vi "Apply IMAQdx Attributes.vi"(8 "error in":errorcluster, 10 "<JSON>":string, 11 "IMAQdx Session in":T1) -> (0 "error out":errorcluster, 3 "Refnum out":T1)   [LabVIEW 2024, in "IMAQdx Base Configure Strategy.lvclass"]
uses:
  IMAQdx Base Configure Strategy.lvclass
  IMAQdx Base Configure Strategy.lvclass/IMAQdx Base Configure Strategy.ctl
  <resource>/objmgr/imaqdx.rc
  <vilib>/JDP Science/JSONtext/JSONtext.lvlib
  <vilib>/Utility/error.llb/whitespace.ctl
  <vilib>/userDefined/High Color/IMAQdx.ctl
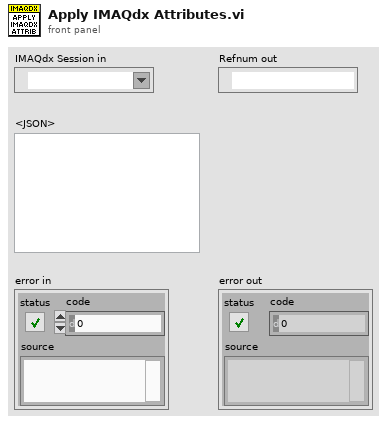
[diagram p1: front panel]
types:
  T1 = typedef "IMAQdx.ctl" = refnum<k21>
  T2 = typedef "JSONtext.lvlib/JSON Value Type.ctl" = enum16{"Not a JSON Value", "JSON Object", "JSON Array", "String", "Number", "true", "false", "null"}
  T3 = typedef "whitespace.ctl" = u16
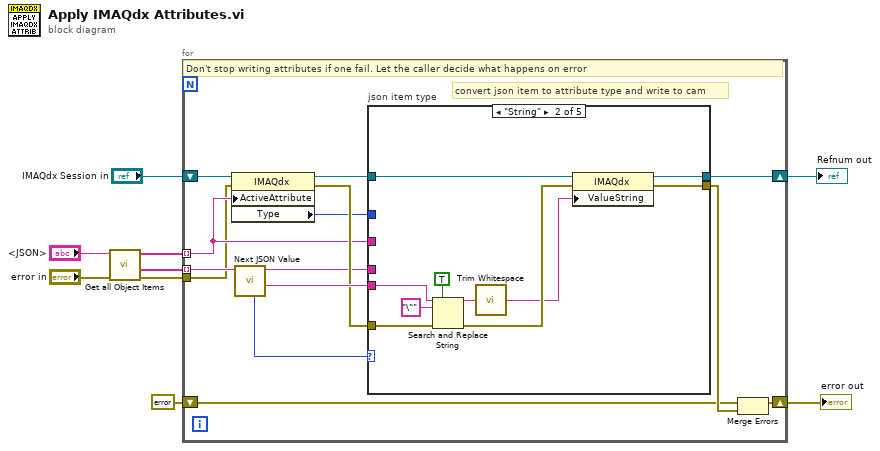
[diagram p0: block diagram]
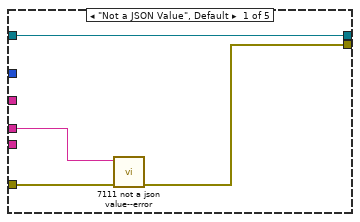
[diagram p2: hidden frame]
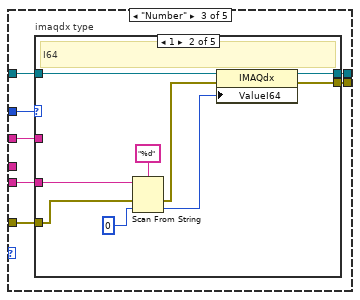
[diagram p3: hidden frame]
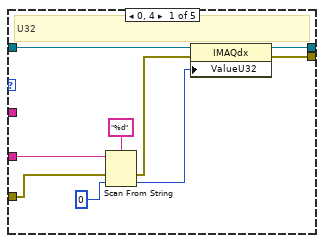
[diagram p4: hidden frame]
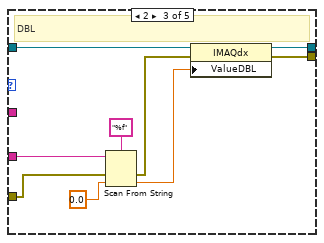
[diagram p5: hidden frame]
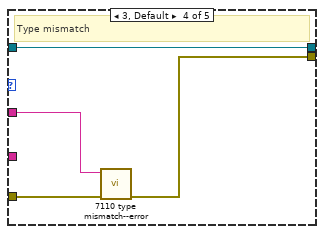
[diagram p6: hidden frame]
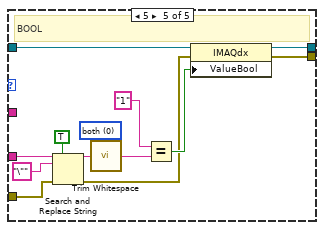
[diagram p7: hidden frame]
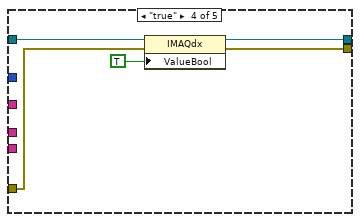
[diagram p8: hidden frame]
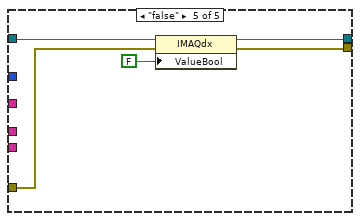
[diagram p9: hidden frame]
diagram:
  n1 = call <vilib>:"Get all Object Items.vi"("error in (no error)"="error in", "JSON"="<JSON>") -> ("error out"=w5:errorcluster, "<JSON>"=w3:string[], "Item Names"=w6:string[])  [unwired: 6 in, 1 out]
  n2 = for {
    shift-right: [w21] -> w9
    shift-left: "IMAQdx Session in" -> [w23]
    tunnel: w6 -> [w15] mode=indexing
    tunnel: w3 -> [w20] mode=indexing
    shift-right: [w11] -> w1
    shift-left: errorcluster {"status"=FALSE, "code"=0, "source"=""} ("error out") -> [w10]
    tunnel: w5 -> [w12]
    # "convert json item to attribute type and write to cam"
    # "Don't stop writing attributes if one fail. Let the caller decide what happens on error"
    n3 = property class="IMAQdx"(reference=w23, error in=w12, "ActiveAttribute"=w15) -> (reference out=w22:T1, error out=w18:errorcluster, "Type"=w17:u32)
    n4 = call <vilib>:"Next JSON Value.vi"("JSON"=w20) -> ("<JSON>"=w19:string, "Rest of Input String"=w14:string, "JSON Value Type"=w16:T2)  [unwired: 7 in, 1 out]
    n5 = case "json item type" shown="\"String\"" w16 {
      tunnel: w22 -> [w24 w37 w44 w91 w97]
      tunnel: [w24 w35 w38 w90 w94] -> w21
      tunnel: w19 -> [_ w34 w43 _ _]
      tunnel: w18 -> [w27 w33 w42 w93 w96]
      tunnel: w17 -> [_ _ w41 _ _]
      tunnel: [w26 w36 w40 w92 w95] -> w13
      tunnel: w15 -> [_ _ w39 _ _]
      tunnel: w14 -> [w25 _ _ _ _]
      frame "Not a JSON Value", Default {
        n6 = call "7111 not a json value--error.vi"("error in"=w27, "Argument"=w25) -> ("error out"=w26:errorcluster)  [unwired: 9 in]
      }
      frame "String" {
        n7 = Search and Replace String(replace all?=TRUE ("replace all? (F)"), input string=w34, search string="\"", error in=w33) -> (result string=w30:string, error out=w32:errorcluster)  [unwired: 4 in, 2 out]
        n8 = call <vilib>:"Trim Whitespace.vi"("string"=w30) -> ("trimmed string"=w29:string)  [unwired: 1 in]
        n9 = property class="IMAQdx"(reference=w37, error in=w32, "ValueString"=w29) -> (reference out=w35:T1, error out=w36:errorcluster)
      }
      frame "Number" {
        n10 = case "imaqdx type" shown="1" w41 {
          tunnel: w44 -> [w49 w58 w67 w72 w84]
          tunnel: w42 -> [w51 w60 w69 w75 w85]
          tunnel: w43 -> [w53 w62 w71 _ w88]
          tunnel: [w46 w55 w64 w74 w83] -> w40
          tunnel: w39 -> [_ _ _ w73 _]
          tunnel: [w45 w54 w63 w72 w82] -> w38
          frame 0, 4 {
            # "U32"
            n11 = Scan From String(format string="%d", input string=w53, error in=w51, default 1=u32 0) -> (error out=w47:errorcluster, output 1=w48:u32)  [unwired: 1 in, 2 out]
            n12 = property class="IMAQdx"(reference=w49, error in=w47, "ValueU32"=w48) -> (reference out=w45:T1, error out=w46:errorcluster)
          }
          frame 1 {
            # "I64"
            n13 = Scan From String(format string="%d", input string=w62, error in=w60, default 1=i64 0) -> (error out=w56:errorcluster, output 1=w57:i64)  [unwired: 1 in, 2 out]
            n14 = property class="IMAQdx"(reference=w58, error in=w56, "ValueI64"=w57) -> (reference out=w54:T1, error out=w55:errorcluster)
          }
          frame 2 {
            # "DBL"
            n15 = Scan From String(format string="%f", input string=w71, error in=w69, default 1=0.0) -> (error out=w65:errorcluster, output 1=w66:dbl)  [unwired: 1 in, 2 out]
            n16 = property class="IMAQdx"(reference=w67, error in=w65, "ValueDBL"=w66) -> (reference out=w63:T1, error out=w64:errorcluster)
          }
          frame 3, Default {
            # "Type mismatch"
            n17 = call "7110 type mismatch--error.vi"("error in"=w75, "Argument"=w73) -> ("error out"=w74:errorcluster)  [unwired: 9 in]
          }
          frame 5 {
            w80 = T3 0 items=["both", "start of string", "end of string"] ("location (both)")
            # "BOOL"
            n18 = Search and Replace String(replace all?=TRUE ("replace all? (F)"), input string=w88, search string="\"", error in=w85) -> (result string=w81:string, error out=w78:errorcluster)  [unwired: 4 in, 2 out]
            n19 = call <vilib>:"Trim Whitespace.vi"("string"=w81, "location (both)"=w80) -> ("trimmed string"=w76:string)
            n20 = Equal?(x="1", y=w76) -> (x = y?=w79:bool)
            n21 = property class="IMAQdx"(reference=w84, error in=w78, "ValueBool"=w79) -> (reference out=w82:T1, error out=w83:errorcluster)
          }
        }
      }
      frame "true" {
        n22 = property class="IMAQdx"(reference=w91, error in=w93, "ValueBool"=TRUE) -> (reference out=w90:T1, error out=w92:errorcluster)
      }
      frame "false" {
        n23 = property class="IMAQdx"(reference=w97, error in=w96, "ValueBool"=FALSE) -> (reference out=w94:T1, error out=w95:errorcluster)
      }
    }
    n24 = Merge Errors(w10, w13) -> (w11:errorcluster)
  }
  "error out" <- w1
  "Refnum out" <- w9
